vi "Finish.vi"   [LabVIEW 2017]
doc: "This VI is called just before exiting. It is expected to close I/O refnum, save collected data, etc."
uses:
  <vilib>/Rock Robotics/WPI/Utilities/WPI_GetSetVariantRefNum.vi
  <vilib>/Rock Robotics/WPI/Ultrasonic/WPI_SonarSRF04DigitalRefNum Registry Get.vi
  <vilib>/Rock Robotics/WPI/Ultrasonic/WPI_SonarSRF04DigitalClose.vi
types:
  T1 = typedef "WPI_UltrasonicDeviceRef.ctl" = cluster{"DevStatus":errorcluster, "Ping Channel":T2, "Echo Channel":T2, "CntIndex":T3}
  T2 = typedef "FPGA_DIOChannel.ctl" = enum8{"DIO 0", "DIO 1", "DIO 2", "DIO 3", "DIO 4", "DIO 5", "DIO 6", "DIO 7", "DIO 8", "DIO 9", "DIO MXP 0", "DIO MXP 1", "DIO MXP 2", "DIO MXP 3", "DIO MXP 4", "DIO MXP 5", "DIO MXP 6", "DIO MXP 7", "DIO MXP 8", "DIO MXP 9", "DIO MXP 10", "DIO MXP 11", "DIO MXP 12", "DIO MXP 13", "DIO MXP 14", "DIO MXP 15", "SPI Port CS1", "SPI Port CS2", "SPI Port CS3", "SPI Port MISO", "SPI Port MOSI", "Invalid"}
  T3 = typedef "FPGA_CounterCtrSystemIndex.ctl" = enum8{"Ctr 0", "Ctr 1", "Ctr 2", "Ctr 3", "Ctr 4", "Ctr 5", "Ctr 6", "Ctr 7", "Invalid"}
  T4 = typedef "WPI_JoystickDevRef.ctl" = cluster{"Device":T5}
  T5 = typedef "WPI_JoystickDeviceEnum.ctl" = enum16{"USB 0", "USB 1", "USB 2", "USB 3", "USB 4", "USB 5"}
  T6 = typedef "WPI_SwitchDevRef.ctl" = cluster{"DevStatus":errorcluster, "DIO Channel":T2, "CntIndex":T3, "Normally Closed":bool}
  T7 = typedef "WPI_MotorControlDeviceRef.ctl" = cluster{"DeviceStatus":errorcluster, "Type":T8, "PWM":cluster{"PWM Channel":T9, "DeadBand":T10}, "CAN":cluster{"Device Number":u8, "SetOutput VI Ref":variant, "GetOutput VI Ref":variant, "Enable VI Ref":variant, "Disable VI Ref":variant, "Data":variant}, "Invert":bool, "DIO PWM":cluster{"PWM \"Enable\" Channel":T9, "DIOChannel":T2, "PWM Rate":dbl}}
  T8 = typedef "WPI_MotorControlType.ctl" = enum16{"PWM", "CAN", "DIO PWM"}
  T9 = typedef "FPGA_DIOPWMChannel.ctl" = enum8{"PWM 0", "PWM 1", "PWM 2", "PWM 3", "PWM 4", "PWM 5", "PWM 6", "PWM 7", "PWM 8", "PWM 9", "PWM MXP 0", "PWM MXP 1", "PWM MXP 2", "PWM MXP 3", "PWM MXP 4", "PWM MXP 5", "PWM MXP 6", "PWM MXP 7", "PWM MXP 8", "PWM MXP 9", "Invalid"}
  T10 = typedef "WPI_PWMDeadband.ctl" = cluster{"Name":string, "maxPositivePwm":i32, "minPositivePwm":i32, "centerPwm":i32, "maxNegativePwm":i32, "minNegativePwm":i32, "angularRange":u16}
  T11 = typedef "WPI_SolenoidDevRef.ctl" = cluster{"DevStatus":errorcluster, "Pneumatics Control Module":u8, "Forward Solenoid Channel":T12, "Reverse Solenoid Channel":T12}
  T12 = typedef "WPI_SolenoidChannel.ctl" = enum8{"Solenoid 0", "Solenoid 1", "Solenoid 2", "Solenoid 3", "Solenoid 4", "Solenoid 5", "Solenoid 6", "Solenoid 7", "Invalid"}
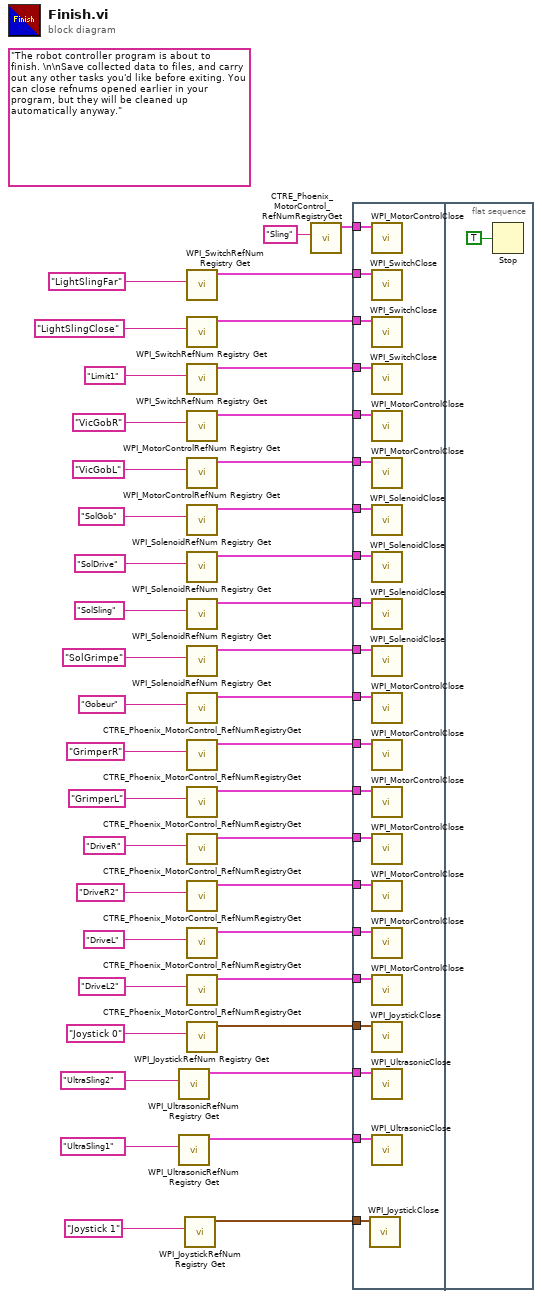
[diagram p0: block diagram]
diagram:
  (unwired) "The robot controller program is about to finish. \n\nSave collected data to files, and carry out any other tasks you'd like before exiting. You can close refnums opened earlier in your program, but they will be cleaned up automatically anyway."
  n1 = call-poly <vilib>:"WPI_UltrasonicRefNum Registry Get.vi"("refnum name"="UltraSling2") -> ("SonarSRF04DevRef"=w21:T1)  [unwired: 9 in, 1 out]
  n2 = call-poly <vilib>:"WPI_UltrasonicRefNum Registry Get.vi"("refnum name"="UltraSling1") -> ("SonarSRF04DevRef"=w24:T1)  [unwired: 9 in, 1 out]
  n3 = call <vilib>:"WPI_JoystickRefNum Registry Get.vi"("refnum name"="Joystick 1") -> ("JoystickDevRef"=w2:T4)  [unwired: 1 in, 9 out]
  n4 = call <vilib>:"WPI_SwitchRefNum Registry Get.vi"("refnum name"="LightSlingFar") -> ("SwitchDevRef"=w18:T6)  [unwired: 9 in, 1 out]
  n5 = call <vilib>:"WPI_SwitchRefNum Registry Get.vi"("refnum name"="LightSlingClose") -> ("SwitchDevRef"=w19:T6)  [unwired: 9 in, 1 out]
  n6 = call <vilib>:"WPI_SwitchRefNum Registry Get.vi"("refnum name"="Limit1") -> ("SwitchDevRef"=w20:T6)  [unwired: 9 in, 1 out]
  n7 = call <vilib>:"WPI_MotorControlRefNum Registry Get.vi"("refnum name"="VicGobR") -> ("MotorControlDevRef"=w5:T7)  [unwired: 9 in, 1 out]
  n8 = call <vilib>:"WPI_MotorControlRefNum Registry Get.vi"("refnum name"="VicGobL") -> ("MotorControlDevRef"=w6:T7)  [unwired: 9 in, 1 out]
  n9 = call <vilib>:"WPI_SolenoidRefNum Registry Get.vi"("refnum name"="SolGob") -> ("SolenoidDevRef"=w11:T11)  [unwired: 9 in, 1 out]
  n10 = call <vilib>:"WPI_SolenoidRefNum Registry Get.vi"("refnum name"="SolDrive") -> ("SolenoidDevRef"=w12:T11)  [unwired: 9 in, 1 out]
  n11 = call <vilib>:"WPI_SolenoidRefNum Registry Get.vi"("refnum name"="SolSling") -> ("SolenoidDevRef"=w13:T11)  [unwired: 9 in, 1 out]
  n12 = call <vilib>:"WPI_SolenoidRefNum Registry Get.vi"("refnum name"="SolGrimpe") -> ("SolenoidDevRef"=w14:T11)  [unwired: 9 in, 1 out]
  n13 = call "CTRE_Phoenix_MotorControl_RefNumRegistryGet.vi"("refnum name"="Gobeur") -> ("PhoenixMotorControlDevRef"=w25:T7)  [unwired: 9 in, 1 out]
  n14 = call "CTRE_Phoenix_MotorControl_RefNumRegistryGet.vi"("refnum name"="GrimperR") -> ("PhoenixMotorControlDevRef"=w26:T7)  [unwired: 9 in, 1 out]
  n15 = call "CTRE_Phoenix_MotorControl_RefNumRegistryGet.vi"("refnum name"="GrimperL") -> ("PhoenixMotorControlDevRef"=w27:T7)  [unwired: 9 in, 1 out]
  n16 = call "CTRE_Phoenix_MotorControl_RefNumRegistryGet.vi"("refnum name"="DriveR") -> ("PhoenixMotorControlDevRef"=w29:T7)  [unwired: 9 in, 1 out]
  n17 = call "CTRE_Phoenix_MotorControl_RefNumRegistryGet.vi"("refnum name"="DriveR2") -> ("PhoenixMotorControlDevRef"=w30:T7)  [unwired: 9 in, 1 out]
  n18 = call "CTRE_Phoenix_MotorControl_RefNumRegistryGet.vi"("refnum name"="DriveL") -> ("PhoenixMotorControlDevRef"=w31:T7)  [unwired: 9 in, 1 out]
  n19 = call "CTRE_Phoenix_MotorControl_RefNumRegistryGet.vi"("refnum name"="DriveL2") -> ("PhoenixMotorControlDevRef"=w40:T7)  [unwired: 9 in, 1 out]
  n20 = call <vilib>:"WPI_JoystickRefNum Registry Get.vi"("refnum name"="Joystick 0") -> ("JoystickDevRef"=w41:T4)  [unwired: 1 in, 9 out]
  n21 = call "CTRE_Phoenix_MotorControl_RefNumRegistryGet.vi"("refnum name"="Sling") -> ("PhoenixMotorControlDevRef"=w28:T7)  [unwired: 9 in, 1 out]
  n22 = flat-sequence {
    tunnel: w41 -> [w63]
    tunnel: w40 -> [w62]
    tunnel: w31 -> [w61]
    tunnel: w30 -> [w60]
    tunnel: w29 -> [w59]
    tunnel: w28 -> [w58]
    tunnel: w27 -> [w57]
    tunnel: w26 -> [w56]
    tunnel: w25 -> [w55]
    tunnel: w24 -> [w54]
    tunnel: w21 -> [w53]
    tunnel: w20 -> [w52]
    tunnel: w19 -> [w51]
    tunnel: w18 -> [w50]
    tunnel: w14 -> [w49]
    tunnel: w13 -> [w48]
    tunnel: w12 -> [w47]
    tunnel: w11 -> [w46]
    tunnel: w6 -> [w45]
    tunnel: w5 -> [w44]
    tunnel: w2 -> [w43]
    frame #0 {
      n23 = call <vilib>:"WPI_JoystickClose.vi"("JoystickDevRef"=w43) -> ()  [unwired: 11 out]
      n24 = call <vilib>:"WPI_MotorControlClose.vi"("MotorControlDevRef"=w58) -> ()  [unwired: 10 in, 1 out]
      n25 = call <vilib>:"WPI_SwitchClose.vi"("SwitchDevRef"=w50) -> ()  [unwired: 10 in, 1 out]
      n26 = call <vilib>:"WPI_SwitchClose.vi"("SwitchDevRef"=w51) -> ()  [unwired: 10 in, 1 out]
      n27 = call <vilib>:"WPI_SwitchClose.vi"("SwitchDevRef"=w52) -> ()  [unwired: 10 in, 1 out]
      n28 = call <vilib>:"WPI_MotorControlClose.vi"("MotorControlDevRef"=w44) -> ()  [unwired: 10 in, 1 out]
      n29 = call <vilib>:"WPI_MotorControlClose.vi"("MotorControlDevRef"=w45) -> ()  [unwired: 10 in, 1 out]
      n30 = call <vilib>:"WPI_SolenoidClose.vi"("SolenoidDevRef"=w46) -> ()  [unwired: 10 in, 1 out]
      n31 = call <vilib>:"WPI_SolenoidClose.vi"("SolenoidDevRef"=w47) -> ()  [unwired: 10 in, 1 out]
      n32 = call <vilib>:"WPI_SolenoidClose.vi"("SolenoidDevRef"=w48) -> ()  [unwired: 10 in, 1 out]
      n33 = call <vilib>:"WPI_SolenoidClose.vi"("SolenoidDevRef"=w49) -> ()  [unwired: 10 in, 1 out]
      n34 = call <vilib>:"WPI_MotorControlClose.vi"("MotorControlDevRef"=w55) -> ()  [unwired: 10 in, 1 out]
      n35 = call <vilib>:"WPI_MotorControlClose.vi"("MotorControlDevRef"=w56) -> ()  [unwired: 10 in, 1 out]
      n36 = call <vilib>:"WPI_MotorControlClose.vi"("MotorControlDevRef"=w57) -> ()  [unwired: 10 in, 1 out]
      n37 = call <vilib>:"WPI_MotorControlClose.vi"("MotorControlDevRef"=w59) -> ()  [unwired: 10 in, 1 out]
      n38 = call <vilib>:"WPI_MotorControlClose.vi"("MotorControlDevRef"=w60) -> ()  [unwired: 10 in, 1 out]
      n39 = call <vilib>:"WPI_MotorControlClose.vi"("MotorControlDevRef"=w61) -> ()  [unwired: 10 in, 1 out]
      n40 = call <vilib>:"WPI_MotorControlClose.vi"("MotorControlDevRef"=w62) -> ()  [unwired: 10 in, 1 out]
      n41 = call <vilib>:"WPI_JoystickClose.vi"("JoystickDevRef"=w63) -> ()  [unwired: 11 out]
      n42 = call-poly <vilib>:"WPI_UltrasonicClose.vi"("SonarSRF04DevRef"=w53) -> ()  [unwired: 10 in, 1 out]
      n43 = call-poly <vilib>:"WPI_UltrasonicClose.vi"("SonarSRF04DevRef"=w54) -> ()  [unwired: 10 in, 1 out]
    }
    frame #1 {
      n44 = Stop(stop? (T)=TRUE ("Quit")) -> ()
    }
  }
